vi "ATS_Acquire.vi"(8 "error in (no error)":errorcluster, 10 "Array":u16[](array[numeric]), 11 "Handle in":u32) -> (0 "error out":errorcluster, 1 "Return Code":u32, 2 "Handle":u32, 3 "Buffer":u16[](array[numeric]))   [LabVIEW 2016]
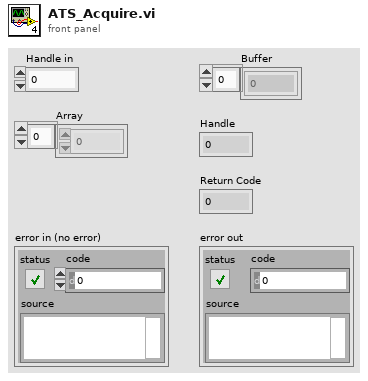
[diagram p1: front panel]
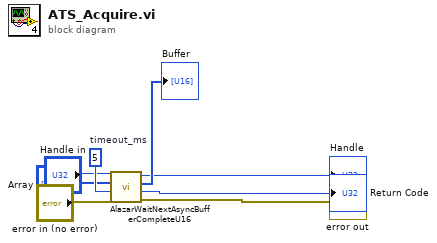
[diagram p0: block diagram]
diagram:
  w3 = u32 5  # timeout_ms
  n1 = call "AlazarWaitNextAsyncBufferCompleteU16.vi"("error in (no error)"="error in (no error)", "timeout_ms"=w3, "Buffer"="Array", "Handle"="Handle in") -> ("error out"=→"error out":errorcluster, "Return Code"=→"Return Code":u32, "Buffer"=→"Buffer":u16[], "Handle"=→"Handle":u32)
